vi "Construct Voltage.vi"(8 "error in (no error)":errorcluster, 9 "Slew":dbl, 10 "Voltage":dbl, 11 "VISA resource name":refnum<visa-resource-name>) -> (0 "error out":errorcluster, 3 "VISA resource name out":refnum<visa-resource-name>)   [LabVIEW 2019, in "7976A.lvlib" / "7976A.lvclass"]
uses:
  Library/7976A.lvclass
  <instrlib>/Agilent N7976A/Agilent N7976A.lvlib
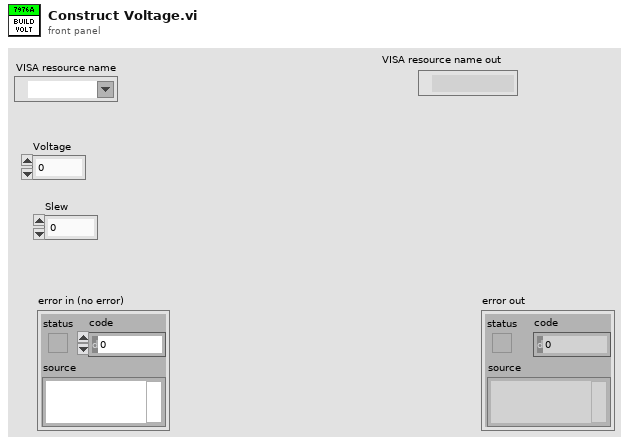
[diagram p1: front panel]
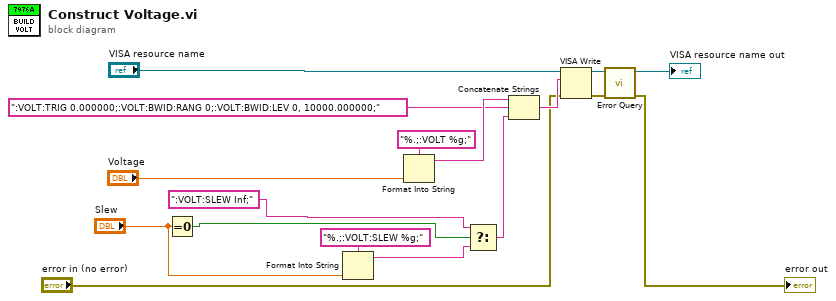
[diagram p0: block diagram]
diagram:
  n1 = Equal To 0?(x="Slew") -> (x = 0?=w6:bool)
  n2 = Format Into String(format string="%.;:VOLT:SLEW %g;", "Slew") -> (resulting string=w8:string)  [unwired: 2 in, 1 out]
  n3 = Format Into String(format string="%.;:VOLT %g;", "Voltage") -> (resulting string=w13:string)  [unwired: 2 in, 1 out]
  n4 = Select(t=":VOLT:SLEW Inf;" ("format string"), s=w6, f=w8) -> (s? t:f=w9:string)
  n5 = Concatenate Strings(w13, ":VOLT:TRIG 0.000000;:VOLT:BWID:RANG 0;:VOLT:BWID:LEV 0, 10000.000000;" ("string"), w9) -> (w14:string)
  n6 = VISA Write(VISA resource name="VISA resource name", write buffer=w14, error in (no error)="error in (no error)") -> (VISA resource name out=w4:refnum<visa-resource-name>, error out=w3:errorcluster)  [unwired: 1 out]
  n7 = call <instrlib>:"Error Query.vi"("error in (no error)"=w3, "VISA resource name"=w4) -> ("error out"=→"error out":errorcluster, "VISA resource name out"=→"VISA resource name out":refnum<visa-resource-name>)  [unwired: 6 in, 2 out]
